vi "Enum with TypeDef Example.vi"() -> ()   [LabVIEW 2021]
uses:
  Control 22 enum.ctl
panel:
  in  "Enum":T1
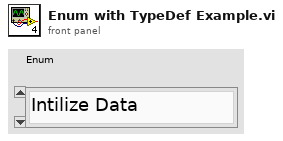
[diagram p1: front panel]
types:
  T1 = typedef "Control 22 enum.ctl" = enum16{"Intilize Data", "Process", "Process 2", "Process 1", "Intilize", "Exit", "MacroExit"}
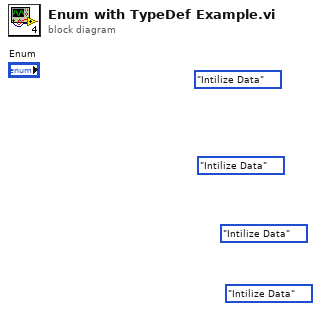
[diagram p0: block diagram]
diagram:
  (unwired) Control_22_enum."Intilize Data" ("Enum")
  (unwired) Control_22_enum."Intilize Data" ("Enum")
  (unwired) Control_22_enum."Intilize Data" ("Enum")
  (unwired) Control_22_enum."Intilize Data" ("Enum")
